vi "ZPL Reset.vi"(6 "Settle (1 mS)":u32=1, 8 "error":errorcluster, 10 "Reset (T)":bool=TRUE, 11 "VISA":refnum<visa-resource-name>) -> (0 "error out":errorcluster, 3 "VISA out":refnum<visa-resource-name>)   [LabVIEW 2015]
doc: "This VI resets the GEN power supply to a known and safe state, if the Reset control is set TRUE (default). This VI will wait for \"Settle\" milliseconds after Reset to allow the output to turn off.\n\nThe reset state includes:\n- Output off\n- Voltage and current program limits to zero\n- Over-voltage protection setting to maximum\n- Under-voltage limit to zero\n- Fold-back protection off\n- Power ON (Autostart) is in off state"
panel:
  # "Lambda ZPLUS \n Serial Port\n  DC Power Supplies"
  # "RESET"
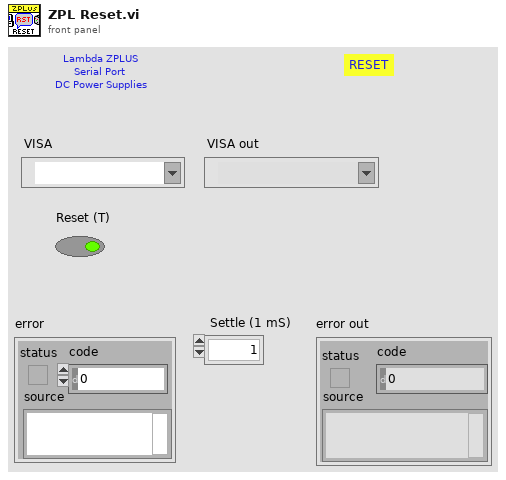
[diagram p1: front panel]
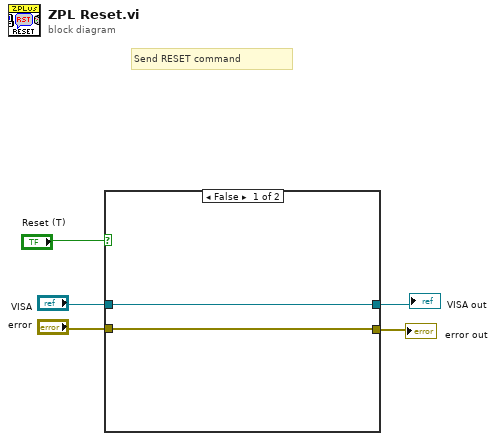
[diagram p0: block diagram]
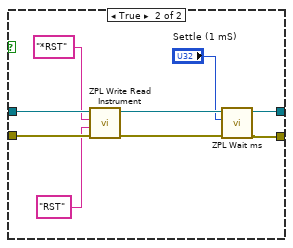
[diagram p2: hidden frame]
diagram:
  # "Send RESET command"
  n1 = case shown="False" "Reset (T)" {
    tunnel: "VISA" -> [w7 w16]
    tunnel: "error" -> [w6 w15]
    tunnel: [w7 w12] -> w3
    tunnel: [w6 w11] -> w2
    frame False {
    }
    frame True {
      n2 = call "ZPL Write Read Instrument.vi"("error in"=w15, "Write Command/Query GEN"="RST", "Write Command/Query SCPI"="*RST", "VISA"=w16) -> ("error out"=w13:errorcluster, "VISA  out"=w14:refnum<visa-resource-name>)  [unwired: 5 in, 1 out]
      n3 = call "ZPL Wait ms.vi"("error"=w13, "Delay (1 mS)"="Settle (1 mS)", "VISA"=w14) -> ("error out"=w11:errorcluster, "VISA out"=w12:refnum<visa-resource-name>)  [unwired: 7 in]
    }
  }
  "error out" <- w2
  "VISA out" <- w3
